vi "IMAQ HL-Sequence.vi"(7 "Skip table":i32[](array[numeric]), 8 "ErrIn":errorcluster, 9 "Number of images":i32=10, 10 "ImgName":string="untitled", 11 "IF Name":string="img0") -> (0 "ErrOut":errorcluster, 3 "ImgOut":T1[](array[typedef]))   [LabVIEW 2013]
doc: "Use this template to build a VI to use as a subVI."
uses:
  <vilib>/vision/Image Controls.llb/IMAQ Image.ctl
panel:
  # "Input Parameters"
  # "Output Parameters"
  # "VI Description:\nThis VI is created to snap a image from imaging device."
  # ":: MVI Framework V1.0 ::\nAuthor:Gaoke Yang\nEmail: gaoke.yang@yahoo.com\nWeb: www.mvicontrol.com\nCopyright (C) 2013, MVI Technologies All Rights Reserved"
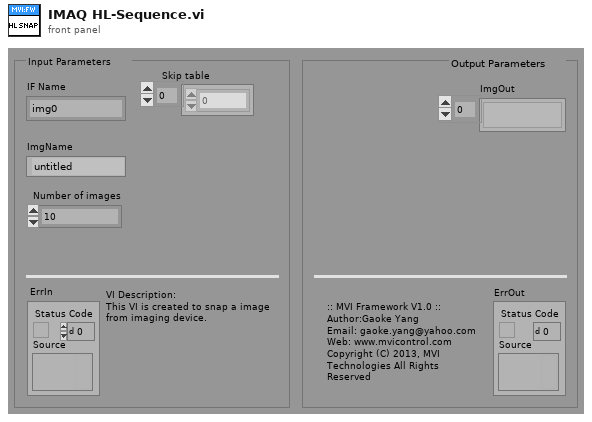
[diagram p1: front panel]
types:
  T1 = typedef "IMAQ Image.ctl" = refnum<image>
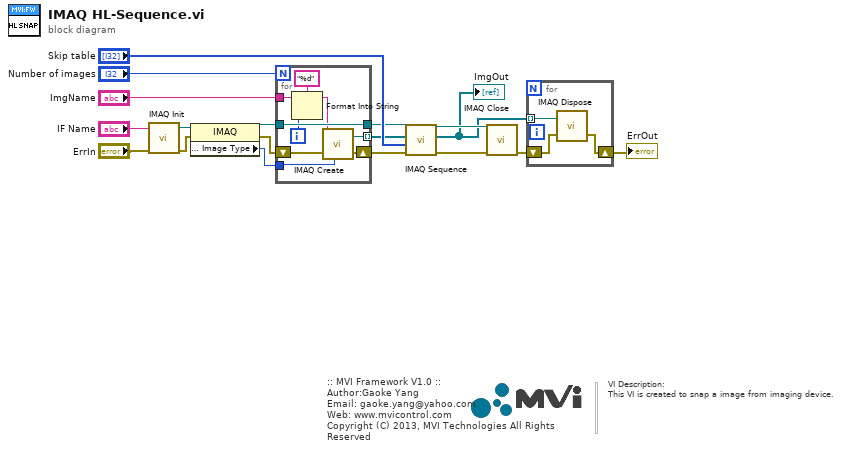
[diagram p0: block diagram]
diagram:
  # "VI Description:\nThis VI is created to snap a image from imaging device."
  # ":: MVI Framework V1.0 ::\nAuthor:Gaoke Yang\nEmail: gaoke.yang@yahoo.com\nWeb: www.mvicontrol.com\nCopyright (C) 2013, MVI Technologies All Rights Reserved"
  n1 = call <vilib>:"IMAQ Init.vi"("error in (no error)"="ErrIn", "Interface Name"="IF Name") -> ("error out"=w8:errorcluster, "IMAQ Session Out"=w9:refnum<k11>)  [unwired: 8 out]
  n2 = property class="IMAQ"(reference=w9, error in=w8) -> (reference out=w6:refnum<k11>, error out=w7:errorcluster, "Image Parameters : Image Type"=w5:u32)
  n3 = for {
    N: "Number of images" -> [_]
    tunnel: [w26] -> w11 mode=indexing
    tunnel: w6 -> [w24]
    tunnel: [w24] -> w12
    tunnel: w5 -> [w23]
    shift-right: [w27] -> w10
    shift-left: w7 -> [w25]
    tunnel: "ImgName" -> [w19]
    i -> [w22]
    n4 = Format Into String(format string="%d", initial string=w19, w22) -> (resulting string=w21:string)  [unwired: 1 in, 1 out]
    n5 = call "IMAQ Create"("Image Name"=w21, "Image Type"=w23, "error in (no error)"=w25) -> ("New Image"=w26:T1, "error out"=w27:errorcluster)  [unwired: 1 in, 1 out]
  }
  n6 = call <vilib>:"IMAQ Sequence.vi"("error in (no error)"=w10, "Skip table"="Skip table", "Images In"=w11, "IMAQ Session In"=w12) -> ("error out"=w3:errorcluster, "Images Out"=w1:T1[], "IMAQ Session Out"=w2:refnum<k11>)  [unwired: 5 out]
  "ImgOut" <- w1
  n7 = call <vilib>:"IMAQ Close.vi"("error in (no error)"=w3, "IMAQ Session In"=w2) -> ("error out"=w4:errorcluster)  [unwired: 9 out]
  n8 = for {
    tunnel: w1 -> [w30] mode=indexing
    shift-right: [w28] -> w14
    shift-left: w4 -> [w29]
    n9 = call "IMAQ Dispose"("Image"=w30, "error in (no error)"=w29) -> ("error out"=w28:errorcluster)  [unwired: 1 in, 3 out]
  }
  "ErrOut" <- w14
